vi "addTestProc.vi"(0 "Config Cluster":T1, 5 "Tree Control":refnum<vi>, 7 "Procedure name":string, 9 "Script name":string, 11 "error in":errorcluster, 12 "Folder to Requirements Documents":path) -> (4 "Config Cluster out":T1, 6 "Tree Control out":refnum<vi>, 15 "error out":errorcluster)   [LabVIEW 2010]
uses:
  Config cluster.ctl
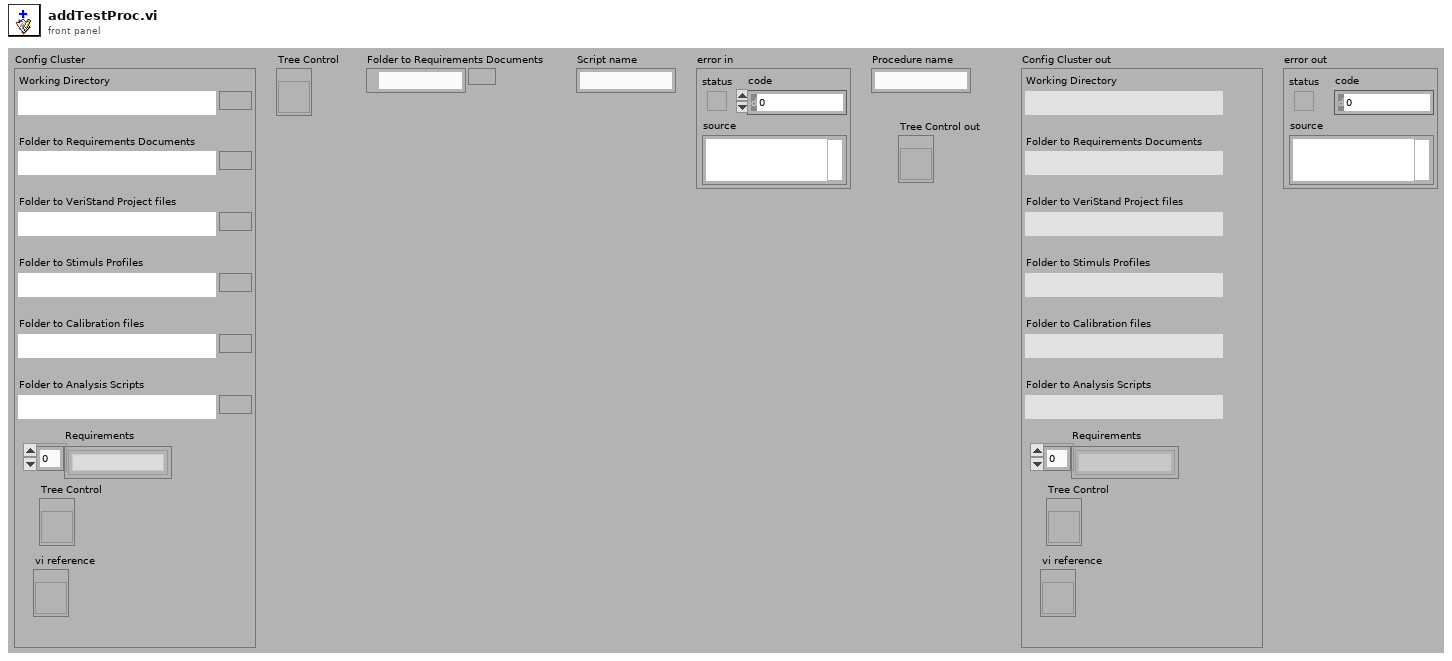
[diagram p1: front panel]
types:
  T1 = typedef "Config cluster.ctl" = cluster{"Working Directory":path, "Folder to Requirements Documents":path, "Folder to VeriStand Project files":path, "Folder to Stimuls Profiles":path, "Folder to Calibration files":path, "Folder to Analysis Scripts":path, "Requirements":string[], "Tree Control":refnum<vi>, "vi reference":refnum<vi>}
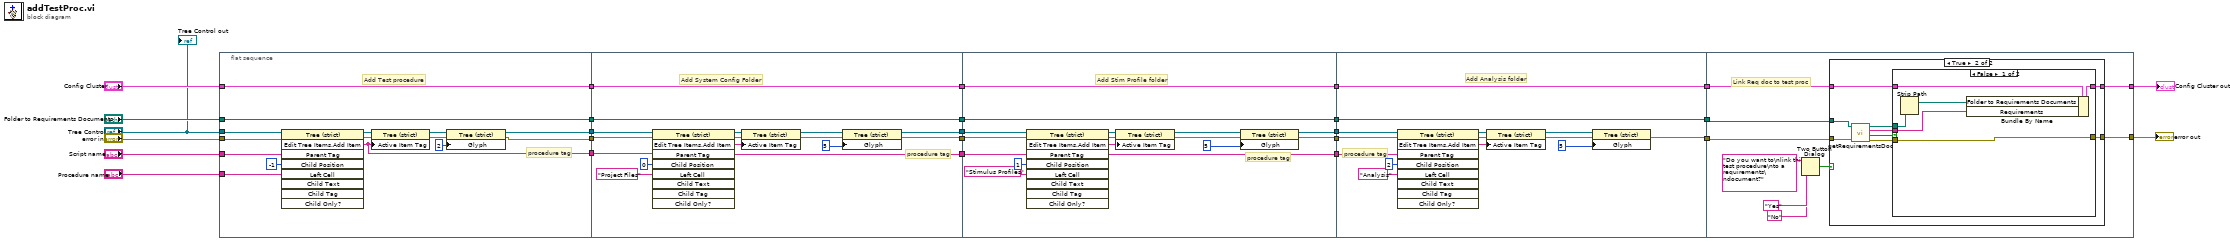
[diagram p0: block diagram]
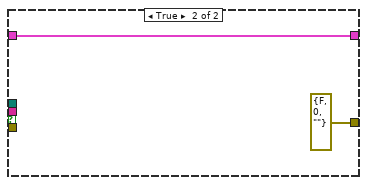
[diagram p3: hidden frame]
diagram:
  n1 = flat-sequence {
    tunnel: "Procedure name" -> [w36]
    tunnel: "Script name" -> [w35]
    tunnel: "Tree Control" -> [w34]
    tunnel: "error in" -> [w32]
    tunnel: [w28] -> w19
    tunnel: "Folder to Requirements Documents" -> [w31]
    tunnel: [w31] -> w18
    tunnel: "Config Cluster" -> [w30]
    tunnel: [w30] -> w17
    tunnel: [w29] -> w16
    tunnel: [w27] -> w2
    tunnel: [w43] -> w15
    tunnel: w19 -> [w47]
    tunnel: [w42] -> w14
    tunnel: w18 -> [w46]
    tunnel: [w46] -> w13
    tunnel: w17 -> [w45]
    tunnel: [w45] -> w12
    tunnel: w16 -> [w44]
    tunnel: [w44] -> w11
    tunnel: w2 -> [w48]
    tunnel: w15 -> [w63]
    tunnel: [w58] -> w10
    tunnel: w14 -> [w62]
    tunnel: [w57] -> w9
    tunnel: w13 -> [w60]
    tunnel: [w60] -> w8
    tunnel: w12 -> [w59]
    tunnel: [w59] -> w7
    tunnel: w11 -> [w61]
    tunnel: [w61] -> w6
    tunnel: w10 -> [w77]
    tunnel: w9 -> [w76]
    tunnel: [w72] -> w5
    tunnel: w8 -> [w74]
    tunnel: [w74] -> w4
    tunnel: w7 -> [w73]
    tunnel: [w73] -> w3
    tunnel: w6 -> [w75]
    tunnel: w5 -> [w91]
    tunnel: w4 -> [w90]
    tunnel: w3 -> [w87]
    tunnel: [w89] -> w26
    tunnel: [w86] -> w1
    frame #0 {
      # "Add Test procedure"
      # "procedure tag"
      n2 = invoke on="Invoke Node" class="Tree (strict)" method="Edit Tree Items.Add Item"(reference=w34, error in=w32, "Parent Tag"=w35, "Child Position"=-1, "Left Cell"=w36) -> (reference out=w39:refnum<vi>, error out=w40:errorcluster, "Edit Tree Items:Add Item"=w29:string)  [unwired: 4 in, 6 out]
      n3 = property on="Property Node" class="Tree (strict)"(reference=w39, error in=w40, "Active Item Tag"=w29) -> (reference out=w38:refnum<vi>, error out=w41:errorcluster)
      n4 = property on="Property Node" class="Tree (strict)"(reference=w38, error in=w41, "Glyph"=2 ("Active Item:Symbol Index")) -> (reference out=w27:refnum<vi>, error out=w28:errorcluster)
    }
    frame #1 {
      # "Add System Config Folder"
      # "procedure tag"
      n5 = invoke on="Invoke Node" class="Tree (strict)" method="Edit Tree Items.Add Item"(reference=w48, error in=w47, "Parent Tag"=w44, "Child Position"=0, "Left Cell"="Project Files" ("Left Cell String")) -> (reference out=w53:refnum<vi>, error out=w54:errorcluster, "Edit Tree Items:Add Item"=w55:string)  [unwired: 4 in, 6 out]
      n6 = property on="Property Node" class="Tree (strict)"(reference=w53, error in=w54, "Active Item Tag"=w55) -> (reference out=w52:refnum<vi>, error out=w56:errorcluster)
      n7 = property on="Property Node" class="Tree (strict)"(reference=w52, error in=w56, "Glyph"=5 ("Active Item:Symbol Index")) -> (reference out=w43:refnum<vi>, error out=w42:errorcluster)
    }
    frame #2 {
      # "Add Stim Profile folder"
      # "procedure tag"
      n8 = invoke on="Invoke Node" class="Tree (strict)" method="Edit Tree Items.Add Item"(reference=w63, error in=w62, "Parent Tag"=w61, "Child Position"=1, "Left Cell"="Stimulus Profiles" ("Left Cell String")) -> (reference out=w68:refnum<vi>, error out=w69:errorcluster, "Edit Tree Items:Add Item"=w70:string)  [unwired: 4 in, 6 out]
      n9 = property on="Property Node" class="Tree (strict)"(reference=w68, error in=w69, "Active Item Tag"=w70) -> (reference out=w67:refnum<vi>, error out=w71:errorcluster)
      n10 = property on="Property Node" class="Tree (strict)"(reference=w67, error in=w71, "Glyph"=5 ("Active Item:Symbol Index")) -> (reference out=w58:refnum<vi>, error out=w57:errorcluster)
    }
    frame #3 {
      # "Add Analysis folder"
      # "procedure tag"
      n11 = invoke on="Invoke Node" class="Tree (strict)" method="Edit Tree Items.Add Item"(reference=w77, error in=w76, "Parent Tag"=w75, "Child Position"=2, "Left Cell"="Analysis" ("Left Cell String")) -> (reference out=w82:refnum<vi>, error out=w83:errorcluster, "Edit Tree Items:Add Item"=w84:string)  [unwired: 4 in, 6 out]
      n12 = property on="Property Node" class="Tree (strict)"(reference=w82, error in=w83, "Active Item Tag"=w84) -> (reference out=w81:refnum<vi>, error out=w85:errorcluster)
      n13 = property on="Property Node" class="Tree (strict)"(reference=w81, error in=w85, "Glyph"=5 ("Active Item:Symbol Index")) -> (error out=w72:errorcluster)  [unwired: 1 out]
    }
    frame #4 {
      # "Link Req doc to test proc"
      n14 = Two Button Dialog(message="Do you want to\nlink this test procedure\nto a requirements\ndocument?", 1:"No" ("F button name (\"Cancel\")"), 2:"Yes" ("T button name (\"OK\")")) -> (T button?=w88:bool)
      n15 = case shown="True" w88 {
        tunnel: w91 -> [w96 w102]
        tunnel: w90 -> [_ w101]
        tunnel: [w96 w104] -> w89
        tunnel: w87 -> [w95 w105]
        tunnel: [w95 w103] -> w86
        frame False {
        }
        frame True {
          n16 = call "getRequirementsDoc.vi"("error in (no error)"=w102, "Path"=w101) -> ("error out"=w99:errorcluster, "Cancelled?"=w100:bool, "Requirements"=w98:string[], "Req Doc Folder"=w97:path)  [unwired: 6 in]
          n17 = case shown="False" w100 {
            tunnel: w105 -> [w111 w113]
            tunnel: [w108 errorcluster {"status"=FALSE, "code"=0, "source"=""} ("error out")] -> w104
            tunnel: [w109 w113] -> w103
            tunnel: w99 -> [w108 _]
            tunnel: w98 -> [w107 _]
            tunnel: w97 -> [w106 _]
            frame False {
              n18 = Strip Path(path=w106) -> (stripped path=w110:path)  [unwired: 1 out]
              n19 = Bundle By Name(cluster=w111, "Folder to Requirements Documents"=w110, "Requirements"=w107) -> (w109:T1)
            }
            frame True {
            }
          }
        }
      }
    }
  }
  "error out" <- w26
  "Config Cluster out" <- w1
  "Tree Control out" <- "Tree Control"
